vi "溶解氧电极校准.vi"() -> ()   [LabVIEW 2016, in "斯坦道多参数.lvlib"]
uses:
  <vilib>/Utility/miscctls.llb/LVPointTypeDef.ctl
  <vilib>/Analysis/NI_AALBase.lvlib
panel:
  out "通讯状态":string
  out "第二点校准值":dbl
  out "第一点校准值":dbl
  out "最小值":sgl format="%#.2f"
  out "最大值":sgl format="%#.2f"
  in  "校准模式":enum16{"两点校准", "单点校准"}(ring)=enum."单点校准"
  in  "校准停止":bool
  in  "校准启动":bool
  out "波形图表":sgl(graph) caption="历史曲线"
  out "变异系数":dbl format="%#.6f"
  out "standard deviation":dbl caption="标准差" format="%#.2f"
  out "mean":dbl caption="均值" format="%#.2f"
  out "测量读值":dbl caption="测量值" format="%#.2f"
  out "偏移值补偿":dbl format="%#.2f"
  out "饱和度值":dbl format="%#.2f"
  out "提示":string
  out "气压补偿值":dbl format="%#.2f"
  out "盐度补偿值":dbl format="%#.2f"
  out "电极斜率":dbl format="%#.6f"
  out "电极零点":dbl format="%#.6f"
  # "溶解氧电极设定"
  # "%"
  # "%"
  # "ppt"
  # "hPa"
  # "mg/L"
  # "请选择校准模式:"
  # "mg/L"
  # "%"
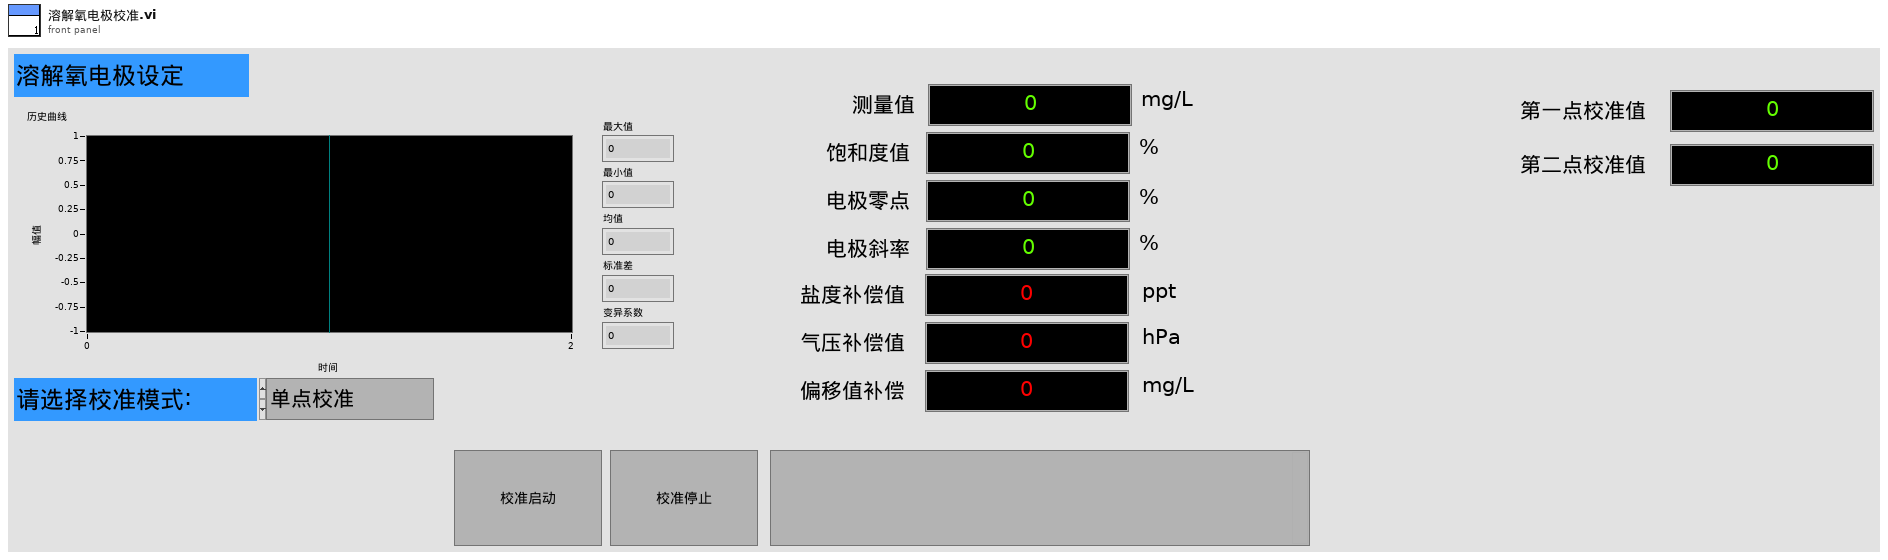
[diagram p1: front panel]
types:
  T1 = typedef "斯坦道多参数.lvlib/校准步骤.ctl" = enum16{"待机", "放置第一点标液", "第一点校准启动", "第一点校准写入", "第一点校准失败", "放置第二点标液", "第二点校准启动", "第二点校准写入", "第二点校准失败", "放置第三点标液", "第三点校准启动", "第三点校准写入", "第三点校准失败", "校准结果写入", "校准结束"}
  T2 = typedef "LVPointTypeDef.ctl" = cluster{"Horizontal":i16, "Vertical":i16}
  T3 = cluster{"电极状态标志":u16, "电极型号标志":u16, "溶解氧测量值":sgl, "温度测量值":sgl, "溶解氧饱和度值":sgl, "盐度补偿值":sgl, "大气压补偿值":sgl, "溶解氧偏移修正值":sgl, "温度偏移修正值":sgl, "手动温度补偿值":sgl, "溶解氧电极零点":sgl, "溶解氧电极斜率":sgl, "第1点标准值记录":sgl, "第1点信号值记录":sgl, "第1点温度值记录":sgl, "第2点标准值记录":sgl, "第2点信号值记录":sgl, "第2点温度值记录":sgl, "命令滤波设定":u16, "温度模式":enum16{"ATC", "MTC"}, "生产批次":u16, "电极序号":u16, "串口地址":u16, "串口波特率":enum16{"9600", "19200", "115200"}, "串口校验位":enum16{"NONE", "ODD", "EVEN"}, "串口停止位":enum16{"1bit", "2bit"}, "第一点标准值":sgl, "第二点标准值":sgl}
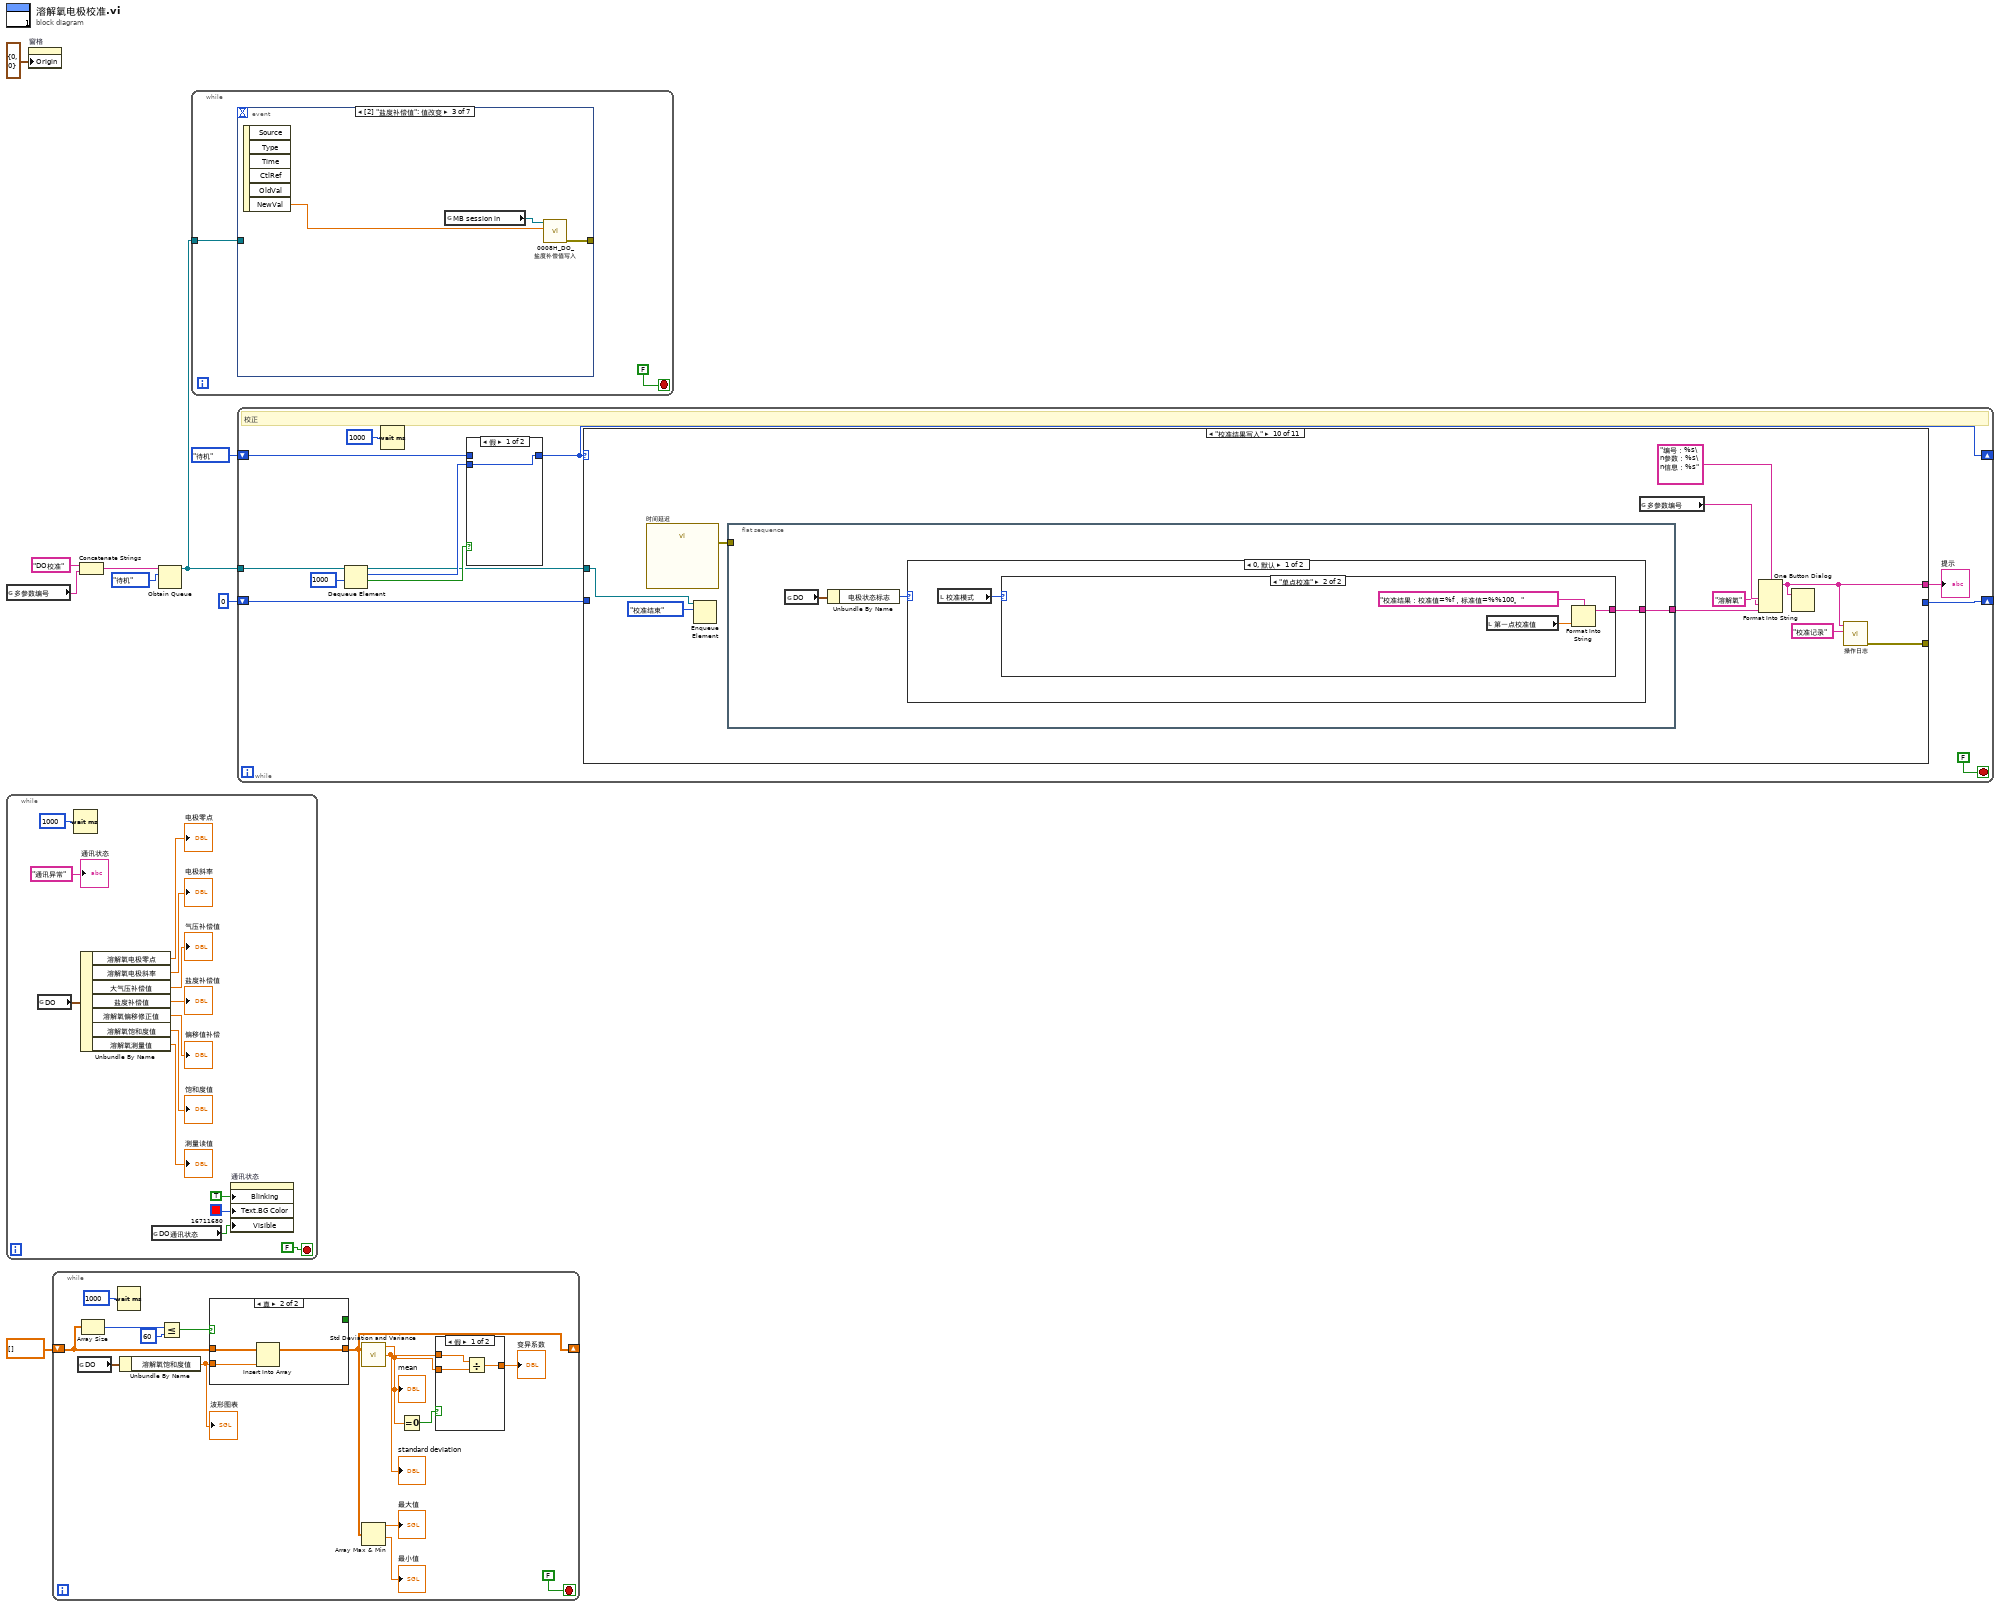
[diagram p0: block diagram]
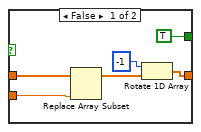
[diagram p3: hidden frame]
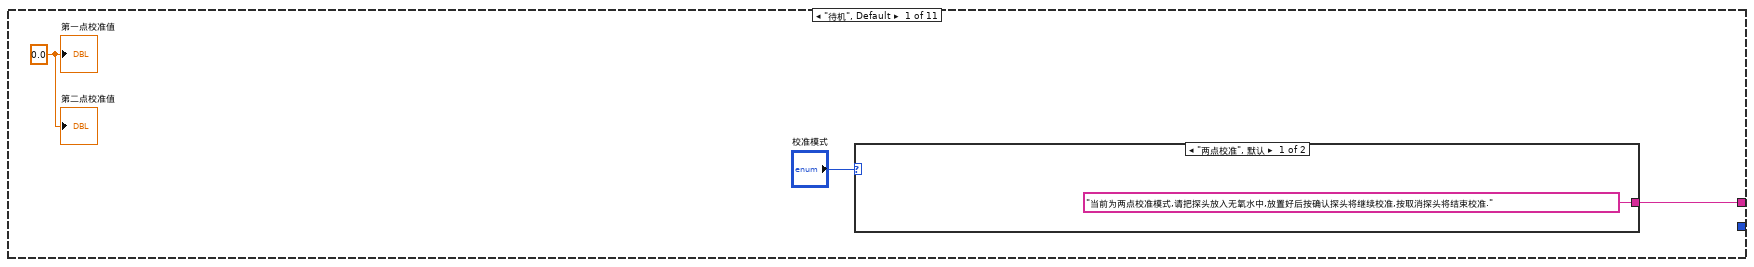
[diagram p5: hidden frame]
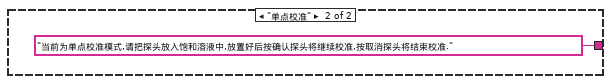
[diagram p6: hidden frame]
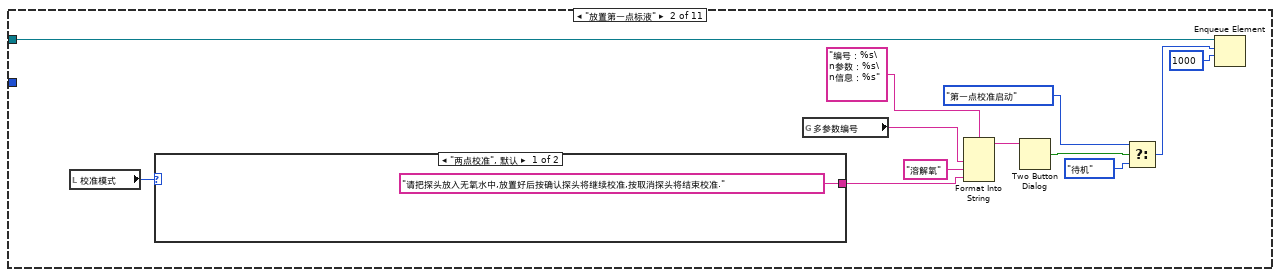
[diagram p7: hidden frame]
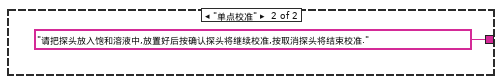
[diagram p8: hidden frame]
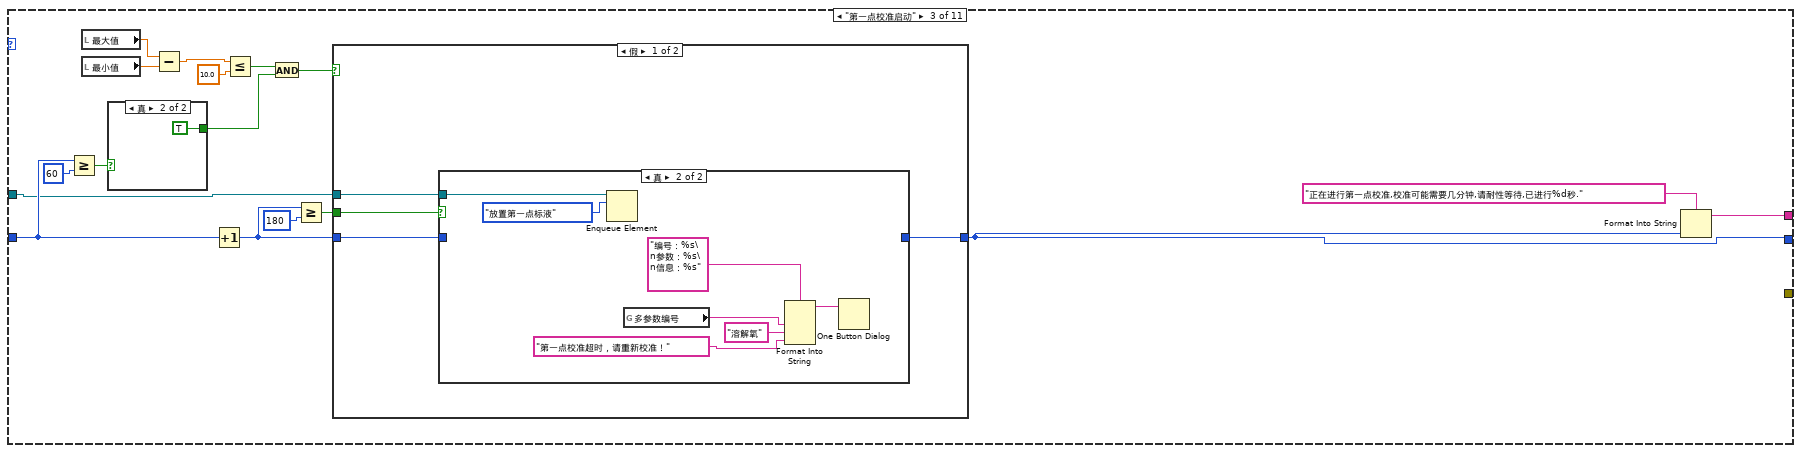
[diagram p9: hidden frame]
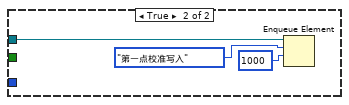
[diagram p11: hidden frame]
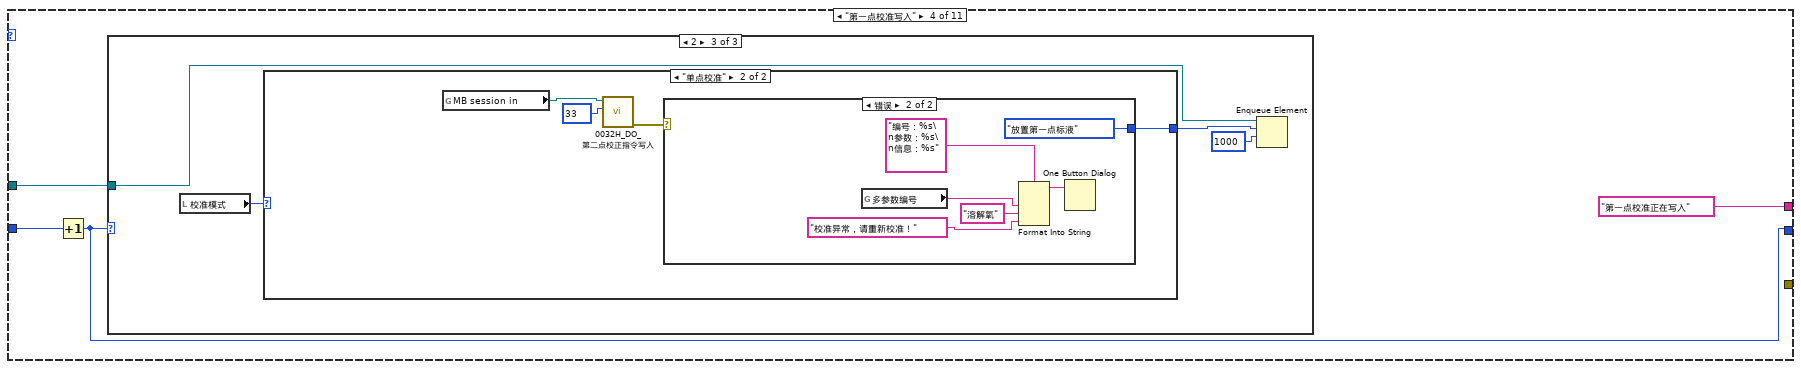
[diagram p13: hidden frame]
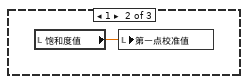
[diagram p15: hidden frame]
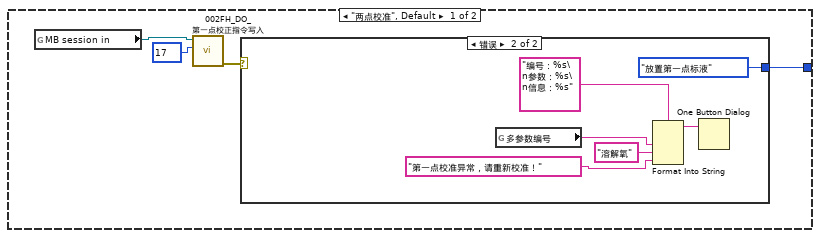
[diagram p16: hidden frame]
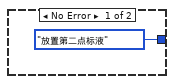
[diagram p17: hidden frame]
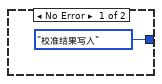
[diagram p18: hidden frame]
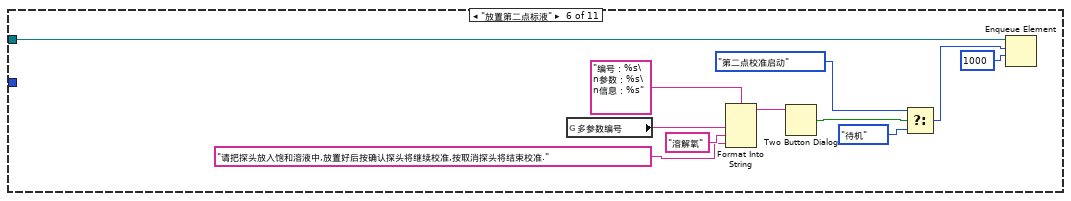
[diagram p20: hidden frame]
diagram:
  n1 = global read "多参数全局变量.vi" "多参数编号"() -> (w1:string)
  n2 = while {
    stop <- FALSE stop-if-true
    n3 = global read "国弘过程全局变量.vi" "DO"() -> (w21:T3)
    n4 = Wait (ms)(milliseconds to wait=u32 1000 ("等待时间（毫秒）")) -> ()  [unwired: 1 out]
    n5 = Unbundle By Name(w21) -> ("溶解氧电极零点"=→"电极零点":sgl, "溶解氧电极斜率"=→"电极斜率":sgl, "大气压补偿值"=→"气压补偿值":sgl, "盐度补偿值"=→"盐度补偿值":sgl, "溶解氧偏移修正值"=→"偏移值补偿":sgl, "溶解氧饱和度值"=→"饱和度值":sgl, "溶解氧测量值"=→"测量读值":sgl)
    n6 = global read "多参数全局变量.vi" "DO通讯状态"() -> (w10:bool)
    n7 = property on="通讯状态" class="Str"("Blinking"=TRUE ("闪烁"), "Text.BG Color"=u32 16711680, "Visible"=w10) -> ()  [unwired: 2 in, 2 out]
    "通讯状态" <- "通讯异常" ("当前串口")
  }
  n8 = property on="窗格" class="Pane"("Origin"=T2 {"Horizontal"=0, "Vertical"=0} ("原点")) -> ()  [unwired: 2 in, 2 out]
  n9 = while {
    shift-right: [w27] -> _
    shift-left: sgl[] [] -> [w34]
    stop <- FALSE stop-if-true
    n10 = global read "国弘过程全局变量.vi" "DO"() -> (w30:T3)
    n11 = Array Size(array=w34) -> (size(s)=w36:i32)
    n12 = Wait (ms)(milliseconds to wait=u32 1000 ("等待时间（毫秒）")) -> ()  [unwired: 1 out]
    n13 = Unbundle By Name(w30) -> ("溶解氧饱和度值"=w24:sgl)
    "波形图表" <- w24
    n14 = Less Or Equal?(x=w36, y=60) -> (x <= y?=w35:bool)
    n15 = case shown="真" w35 {
      tunnel: w34 -> [w47 w50]
      tunnel: w24 -> [w45 w49]
      tunnel: [w43 w48] -> w27
      tunnel: [TRUE _] -> _
      frame False {
        n16 = Replace Array Subset(array=w47, new element=w45) -> (w46:sgl[])  [unwired: 1 in]
        n17 = Rotate 1D Array(1:w46, 2:-1 ("n")) -> (0:w43:sgl[])
      }
      frame True {
        n18 = Insert Into Array(array=w50, new element=w49) -> (w48:sgl[])  [unwired: 1 in]
      }
    }
    n19 = call <vilib>:"Std Deviation and Variance.vi"("X"=w27) -> ("mean"=w29:dbl, "standard deviation"=w28:dbl)  [unwired: 1 in, 1 out]
    "mean" <- w29
    "standard deviation" <- w28
    n20 = Array Max & Min(array=w27) -> (max value=→"最大值":sgl, min value=→"最小值":sgl)  [unwired: 2 out]
    n21 = Equal To 0?(x=w29) -> (x = 0?=w33:bool)
    n22 = case shown="假" w33 {
      tunnel: w28 -> [w41 _]
      tunnel: [w40 _] -> w32
      tunnel: w29 -> [w39 _]
      frame False {
        n23 = Divide(x=w41, y=w39) -> (x/y=w40:dbl)
      }
      frame True {
      }
    }
    "变异系数" <- w32
  }
  n24 = Concatenate Strings("DO校准" ("名称（未命名）"), w1) -> (w2:string)
  n25 = Obtain Queue(name (unnamed)=w2, element data type=校准步骤."待机" ("枚举")) -> (queue out=w3:refnum<queue>)  [unwired: 3 in, 2 out]
  n26 = while {
    tunnel: w3 -> [w51]
    stop <- FALSE stop-if-true
    n27 = event shown="[2] \"盐度补偿值\": 值改变" {
      selector: _ -> [_ _ _ _ _ _ _]
      dyn-events: _ -> [_ _ _ _ _ _ _]
      timeout: _ -> [_ _ _ _ _ _ _]
      tunnel: [_ _ w58 w61 w64 _ _] -> _
      tunnel: w51 -> [_ _ _ _ _ w66 w68]
      event Timeout {
        n28 = event-data() -> ()  [unwired: 1 in, 3 out]
      }
      event "盐度补偿值", "气压补偿值", "偏移值补偿": Mouse Down {
        n29 = event-data() -> ("CtlRef"=w54:refnum<vi>)  [unwired: 1 in, 7 out]
        n30 = property class="DigNum (严格)"(reference=w54) -> (reference out=w53:refnum<vi>, "Value"=w55:dbl)  [unwired: 1 in, 1 out]
        n31 = call "数字键盘.vi"("OldNumber"=w55) -> ("NewNumber"=w56:dbl)  [unwired: 1 in]
        n32 = property class="DigNum (严格)"(reference=w53, "Val(Sgnl)"=w56) -> ()  [unwired: 1 in, 2 out]
      }
      event "盐度补偿值": Value Change {
        n33 = event-data() -> ("NewVal"=w59:dbl)  [unwired: 1 in, 5 out]
        n34 = global read "多参数全局变量.vi" "MB session in"() -> (w57:refnum<class "MB_Master.lvclass">)
        n35 = call "0008H_DO_盐度补偿值写入.vi"("数值"=w59, "MB session in"=w57) -> ("error out"=w58:errorcluster)  [unwired: 8 in, 1 out]
      }
      event "气压补偿值": Value Change {
        n36 = event-data() -> ("NewVal"=w62:dbl)  [unwired: 1 in, 5 out]
        n37 = global read "多参数全局变量.vi" "MB session in"() -> (w60:refnum<class "MB_Master.lvclass">)
        n38 = call "000AH_DO_大气压补偿值写入.vi"("数值"=w62, "MB session in"=w60) -> ("error out"=w61:errorcluster)  [unwired: 8 in, 1 out]
      }
      event "偏移值补偿": Value Change {
        n39 = event-data() -> ("NewVal"=w65:dbl)  [unwired: 1 in, 5 out]
        n40 = global read "多参数全局变量.vi" "MB session in"() -> (w63:refnum<class "MB_Master.lvclass">)
        n41 = call "000CH_DO_DO偏移修正值写入.vi"("数值"=w65, "MB session in"=w63) -> ("error out"=w64:errorcluster)  [unwired: 8 in, 1 out]
      }
      event "校准启动": Value Change {
        n42 = event-data() -> ()  [unwired: 1 in, 6 out]
        n43 = Enqueue Element(queue=w66, element=校准步骤."放置第一点标液" ("元素")) -> ()  [unwired: 2 in, 3 out]
      }
      event "校准停止": Value Change {
        n44 = event-data() -> ()  [unwired: 1 in, 6 out]
        n45 = Flush Queue(queue=w68) -> (queue out=w69:refnum<queue>)  [unwired: 1 in, 2 out]
        n46 = Enqueue Element(queue=w69, element=校准步骤."待机" ("元素"), timeout in ms (-1)=1000 ("超时毫秒(-1)")) -> ()  [unwired: 1 in, 3 out]
      }
    }
  }
  n47 = while "While循环" {
    shift-right: [w73] -> _
    shift-left: 校准步骤."待机" ("枚举") -> [w74]
    shift-right: [w80] -> _
    shift-left: 0 -> [w81]
    tunnel: w3 -> [w75]
    stop <- FALSE stop-if-true
    # "校正"
    n48 = Dequeue Element(queue=w75, timeout in ms (-1)=1000 ("超时毫秒(-1)")) -> (queue out=w72:refnum<queue>, element=w76:T1, timed out?=w77:bool)  [unwired: 1 in, 1 out]
    n49 = Wait (ms)(milliseconds to wait=u32 1000 ("等待时间（毫秒）")) -> ()  [unwired: 1 out]
    n50 = case shown="假" w77 {
      tunnel: w76 -> [w84 _]
      tunnel: [w84 w85] -> w73
      tunnel: w74 -> [_ w85]
      frame False {
      }
      frame True {
      }
    }
    n51 = case shown="\"校准结果写入\"" w73 {
      tunnel: [w88 _ w109 "第一点校准正在写入" ("提示") _ _ w181 "第二点校准正在写入" ("提示") _ w233 w257] -> w79
      tunnel: w81 -> [_ _ w113 w140 _ _ w183 w215 _ _ _]
      tunnel: [_ _ w112 w139 _ _ w182 w214 _ _ _] -> w80
      tunnel: w72 -> [_ w97 w111 w138 _ w174 w184 w213 _ w239 _]
      tunnel: [_ _ _ _ _ _ _ _ _ w238 _] -> _
      frame "待机", Default {
        w86 = 0.0 ("第一点校准值")
        n52 = case shown="\"两点校准\", 默认" "校准模式" {
          tunnel: ["当前为两点校准模式,请把探头放入无氧水中,放置好后按确认探头将继续校准,按取消探头将结束校准." ("消息") "当前为单点校准模式,请把探头放入饱和溶液中,放置好后按确认探头将继续校准,按取消探头将结束校准." ("消息")] -> w88
          frame "两点校准", Default {
          }
          frame "单点校准" {
          }
        }
        "第一点校准值" <- w86
        "第二点校准值" <- w86
      }
      frame "放置第一点标液" {
        n53 = local read "校准模式"() -> (w96:enum16{"两点校准", "单点校准"})
        n54 = case shown="\"两点校准\", 默认" w96 {
          tunnel: ["请把探头放入无氧水中,放置好后按确认探头将继续校准,按取消探头将结束校准." ("消息") "请把探头放入饱和溶液中,放置好后按确认探头将继续校准,按取消探头将结束校准." ("消息")] -> w91
          frame "两点校准", Default {
          }
          frame "单点校准" {
          }
        }
        n55 = global read "多参数全局变量.vi" "多参数编号"() -> (w94:string)
        n56 = Format Into String(format string="编号：%s\n参数：%s\n信息：%s" ("格式字符串"), w94, "溶解氧" ("输入 2"), w91) -> (resulting string=w92:string)  [unwired: 2 in, 1 out]
        n57 = Two Button Dialog(message=w92) -> (T button?=w101:bool)  [unwired: 2 in]
        n58 = Select(t=校准步骤."第一点校准启动" ("元素"), s=w101, f=校准步骤."待机" ("元素")) -> (s? t:f=w98:T1)
        n59 = Enqueue Element(queue=w97, element=w98, timeout in ms (-1)=1000 ("超时毫秒(-1)")) -> ()  [unwired: 1 in, 3 out]
      }
      frame "第一点校准启动" {
        n60 = Greater Or Equal?(x=w113, y=60) -> (x >= y?=w120:bool)
        n61 = local read "最大值"() -> (w117:sgl)
        n62 = local read "最小值"() -> (w116:sgl)
        n63 = case shown="真" w120 {
          tunnel: [_ TRUE] -> w108
          frame False {
          }
          frame True {
          }
        }
        n64 = Subtract(x=w117, y=w116) -> (x-y=w118:sgl)
        n65 = Increment(x=w113) -> (x+1=w110:i32)
        n66 = Less Or Equal?(x=w118, y=10.0) -> (x <= y?=w107:bool)
        n67 = And(x=w107, y=w108) -> (x .and. y?=w106:bool)
        n68 = Greater Or Equal?(x=w110, y=180) -> (x >= y?=w114:bool)
        n69 = case shown="假" w106 {
          tunnel: w111 -> [w124 w136]
          tunnel: w114 -> [w125 _]
          tunnel: w110 -> [w123 _]
          tunnel: [w122 _] -> w112
          frame False {
            n70 = case shown="真" w125 {
              tunnel: w124 -> [_ w133]
              tunnel: w123 -> [w126 _]
              tunnel: [w126 _] -> w122
              frame False {
              }
              frame True {
                n71 = Enqueue Element(queue=w133, element=校准步骤."放置第一点标液" ("元素")) -> ()  [unwired: 2 in, 3 out]
                n72 = global read "多参数全局变量.vi" "多参数编号"() -> (w130:string)
                n73 = Format Into String(format string="编号：%s\n参数：%s\n信息：%s" ("格式字符串"), w130, "溶解氧" ("输入 2"), "第一点校准超时，请重新校准！" ("error source (\" \")")) -> (resulting string=w128:string)  [unwired: 2 in, 1 out]
                n74 = One Button Dialog(message=w128) -> ()  [unwired: 1 in, 1 out]
              }
            }
          }
          frame True {
            n75 = Enqueue Element(queue=w136, element=校准步骤."第一点校准写入" ("元素"), timeout in ms (-1)=1000 ("超时毫秒(-1)")) -> ()  [unwired: 1 in, 3 out]
          }
        }
        n76 = Format Into String(format string="正在进行第一点校准,校准可能需要几分钟,请耐性等待,已进行%d秒." ("格式字符串"), w112) -> (resulting string=w109:string)  [unwired: 2 in, 1 out]
      }
      frame "第一点校准写入" {
        n77 = Increment(x=w140) -> (x+1=w139:i32)
        n78 = case shown="2" w139 {
          tunnel: w138 -> [_ _ w144]
          frame 0, Default {
          }
          frame 1 {
            n79 = local read "饱和度值"() -> (w142:dbl)
            n80 = local write "第一点校准值"(w142) -> ()
          }
          frame 2 {
            n81 = local read "校准模式"() -> (w146:enum16{"两点校准", "单点校准"})
            n82 = case shown="\"单点校准\"" w146 {
              tunnel: [w147 w158] -> w143
              frame "两点校准", Default {
                n83 = global read "多参数全局变量.vi" "MB session in"() -> (w148:refnum<class "MB_Master.lvclass">)
                n84 = call "002FH_DO_第一点校正指令写入.vi"("数值"=u16 17, "MB session in"=w148) -> ("error out"=w149:errorcluster)  [unwired: 8 in, 1 out]
                n85 = case shown="错误" w149 {
                  tunnel: [校准步骤."放置第二点标液" ("元素") 校准步骤."放置第一点标液" ("元素")] -> w147
                  frame No Error {
                  }
                  frame Error {
                    n86 = global read "多参数全局变量.vi" "多参数编号"() -> (w155:string)
                    n87 = Format Into String(format string="编号：%s\n参数：%s\n信息：%s" ("格式字符串"), w155, "溶解氧" ("输入 2"), "第一点校准异常，请重新校准！" ("error source (\" \")")) -> (resulting string=w153:string)  [unwired: 2 in, 1 out]
                    n88 = One Button Dialog(message=w153) -> ()  [unwired: 1 in, 1 out]
                  }
                }
              }
              frame "单点校准" {
                n89 = global read "多参数全局变量.vi" "MB session in"() -> (w160:refnum<class "MB_Master.lvclass">)
                n90 = call "0032H_DO_第二点校正指令写入.vi"("数值"=u16 33, "MB session in"=w160) -> ("error out"=w159:errorcluster)  [unwired: 8 in, 1 out]
                n91 = case shown="错误" w159 {
                  tunnel: [校准步骤."校准结果写入" ("元素") 校准步骤."放置第一点标液" ("元素")] -> w158
                  frame No Error {
                  }
                  frame Error {
                    n92 = global read "多参数全局变量.vi" "多参数编号"() -> (w166:string)
                    n93 = Format Into String(format string="编号：%s\n参数：%s\n信息：%s" ("格式字符串"), w166, "溶解氧" ("输入 2"), "校准异常，请重新校准！" ("error source (\" \")")) -> (resulting string=w165:string)  [unwired: 2 in, 1 out]
                    n94 = One Button Dialog(message=w165) -> ()  [unwired: 1 in, 1 out]
                  }
                }
              }
            }
            n95 = Enqueue Element(queue=w144, element=w143, timeout in ms (-1)=1000 ("超时毫秒(-1)")) -> ()  [unwired: 1 in, 3 out]
          }
        }
      }
      frame "第一点校准失败" {
      }
      frame "放置第二点标液" {
        n96 = global read "多参数全局变量.vi" "多参数编号"() -> (w172:string)
        n97 = Format Into String(format string="编号：%s\n参数：%s\n信息：%s" ("格式字符串"), w172, "溶解氧" ("输入 2"), "请把探头放入饱和溶液中,放置好后按确认探头将继续校准,按取消探头将结束校准." ("消息")) -> (resulting string=w169:string)  [unwired: 2 in, 1 out]
        n98 = Two Button Dialog(message=w169) -> (T button?=w178:bool)  [unwired: 2 in]
        n99 = Select(t=校准步骤."第二点校准启动" ("元素"), s=w178, f=校准步骤."待机" ("元素")) -> (s? t:f=w175:T1)
        n100 = Enqueue Element(queue=w174, element=w175, timeout in ms (-1)=1000 ("超时毫秒(-1)")) -> ()  [unwired: 1 in, 3 out]
      }
      frame "第二点校准启动" {
        n101 = Greater Or Equal?(x=w183, y=60) -> (x >= y?=w195:bool)
        n102 = local read "最大值"() -> (w192:sgl)
        n103 = local read "最小值"() -> (w191:sgl)
        n104 = case shown="真" w195 {
          tunnel: [_ TRUE] -> w188
          frame False {
          }
          frame True {
          }
        }
        n105 = Subtract(x=w192, y=w191) -> (x-y=w193:sgl)
        n106 = Increment(x=w183) -> (x+1=w189:i32)
        n107 = Less Or Equal?(x=w193, y=10.0) -> (x <= y?=w187:bool)
        n108 = And(x=w187, y=w188) -> (x .and. y?=w186:bool)
        n109 = Greater Or Equal?(x=w189, y=180) -> (x >= y?=w190:bool)
        n110 = case shown="假" w186 {
          tunnel: w184 -> [w199 w211]
          tunnel: w190 -> [w200 _]
          tunnel: w189 -> [w198 _]
          tunnel: [w197 _] -> w182
          frame False {
            n111 = case shown="真" w200 {
              tunnel: w199 -> [_ w208]
              tunnel: w198 -> [w201 _]
              tunnel: [w201 _] -> w197
              frame False {
              }
              frame True {
                n112 = Enqueue Element(queue=w208, element=校准步骤."放置第二点标液" ("元素")) -> ()  [unwired: 2 in, 3 out]
                n113 = global read "多参数全局变量.vi" "多参数编号"() -> (w205:string)
                n114 = Format Into String(format string="编号：%s\n参数：%s\n信息：%s" ("格式字符串"), w205, "溶解氧" ("输入 2"), "第二点校准超时，请重新校准！" ("error source (\" \")")) -> (resulting string=w203:string)  [unwired: 2 in, 1 out]
                n115 = One Button Dialog(message=w203) -> ()  [unwired: 1 in, 1 out]
              }
            }
          }
          frame True {
            n116 = Enqueue Element(queue=w211, element=校准步骤."第二点校准写入" ("元素"), timeout in ms (-1)=1000 ("超时毫秒(-1)")) -> ()  [unwired: 1 in, 3 out]
          }
        }
        n117 = Format Into String(format string="正在进行第二点校准,校准可能需要几分钟,请耐性等待,已进行%d秒." ("格式字符串"), w182) -> (resulting string=w181:string)  [unwired: 2 in, 1 out]
      }
      frame "第二点校准写入" {
        n118 = Increment(x=w215) -> (x+1=w214:i32)
        n119 = case shown="2" w214 {
          tunnel: w213 -> [_ _ w218]
          frame 0, Default {
            (unwired) 校准步骤."第二点校准写入" ("枚举")
          }
          frame 1 {
            n120 = local read "饱和度值"() -> (w217:dbl)
            n121 = local write "第二点校准值"(w217) -> ()
          }
          frame 2 {
            n122 = global read "多参数全局变量.vi" "MB session in"() -> (w222:refnum<class "MB_Master.lvclass">)
            n123 = call "0032H_DO_第二点校正指令写入.vi"("数值"=u16 33, "MB session in"=w222) -> ("error out"=w219:errorcluster)  [unwired: 8 in, 1 out]
            n124 = case shown="错误" w219 {
              tunnel: [校准步骤."校准结果写入" ("元素") 校准步骤."放置第二点标液" ("元素")] -> w220
              frame No Error {
              }
              frame Error {
                n125 = global read "多参数全局变量.vi" "多参数编号"() -> (w228:string)
                n126 = Format Into String(format string="编号：%s\n参数：%s\n信息：%s" ("格式字符串"), w228, "溶解氧" ("输入 2"), "第二点校准异常，请重新校准！" ("error source (\" \")")) -> (resulting string=w226:string)  [unwired: 2 in, 1 out]
                n127 = One Button Dialog(message=w226) -> ()  [unwired: 1 in, 1 out]
              }
            }
            n128 = Enqueue Element(queue=w218, element=w220, timeout in ms (-1)=1000 ("超时毫秒(-1)")) -> ()  [unwired: 1 in, 3 out]
          }
        }
      }
      frame "第二点校准失败" {
      }
      frame "校准结果写入" {
        n129 = call "时间延迟"() -> ("error out"=w231:errorcluster)  [unwired: 11 in]
        n130 = Enqueue Element(queue=w239, element=校准步骤."校准结束" ("元素")) -> ()  [unwired: 2 in, 3 out]
        n131 = flat-sequence {
          tunnel: [w243] -> w234
          tunnel: w231 -> [_]
          frame #0 {
            n132 = global read "国弘过程全局变量.vi" "DO"() -> (w242:T3)
            n133 = Unbundle By Name(w242) -> ("电极状态标志"=w241:u16)
            n134 = case shown="0, 默认" w241 {
              selector: w241 -> [_ w254]
              tunnel: [w244 w253] -> w243
              frame 0, Default {
                n135 = local read "校准模式"() -> (w245:enum16{"两点校准", "单点校准"})
                n136 = case shown="\"单点校准\"" w245 {
                  tunnel: [w249 w252] -> w244
                  frame "两点校准", Default {
                    n137 = local read "第一点校准值"() -> (w248:dbl)
                    n138 = local read "第二点校准值"() -> (w246:dbl)
                    n139 = Format Into String(format string="校准结果：第一点校准值=%f，第一点标准值=%%0,第二点校准值=%f，第二点标准值=%%100." ("提示"), w248, w246) -> (resulting string=w249:string)  [unwired: 2 in, 1 out]
                  }
                  frame "单点校准" {
                    n140 = local read "第一点校准值"() -> (w251:dbl)
                    n141 = Format Into String(format string="校准结果：校准值=%f，标准值=%%100。" ("提示"), w251) -> (resulting string=w252:string)  [unwired: 2 in, 1 out]
                  }
                }
              }
              frame 3, 4 {
                n142 = case shown="4" w254 {
                  tunnel: ["校正失败，电极零点超出范围" "校正失败，电极斜率超出范围"] -> w253
                  frame 3, Default {
                  }
                  frame 4 {
                  }
                }
              }
            }
          }
        }
        n143 = global read "多参数全局变量.vi" "多参数编号"() -> (w236:string)
        n144 = Format Into String(format string="编号：%s\n参数：%s\n信息：%s" ("格式字符串"), w236, "溶解氧" ("输入 2"), w234) -> (resulting string=w233:string)  [unwired: 2 in, 1 out]
        n145 = One Button Dialog(message=w233) -> ()  [unwired: 1 in, 1 out]
        n146 = call "操作日志.vi"("table"="校准记录", "日志信息"=w233) -> ("error out"=w238:errorcluster)  [unwired: 9 in]
      }
      frame "校准结束" {
        n147 = local read "提示"() -> (w257:string)
      }
    }
    "提示" <- w79
  }
